vi "(SubVI) Cut Unfold and Fold Startpoint_YCC.vi"(7 "number to cut":i32=15, 8 "Folded-Force in":dbl[](array[numeric]), 9 "Folded-xDNA in":dbl[](array[numeric]), 10 "Unfolded-Force":dbl[](array[numeric]), 11 "Unfolded-xDNA":dbl[](array[numeric])) -> (0 "Folded-Force":dbl[](array[numeric]), 1 "Folded-xDNA":dbl[](array[numeric]), 2 "Unfolded-Force":dbl[](array[numeric]), 3 "Unfolded-xDNA":dbl[](array[numeric]))   [LabVIEW 2014]
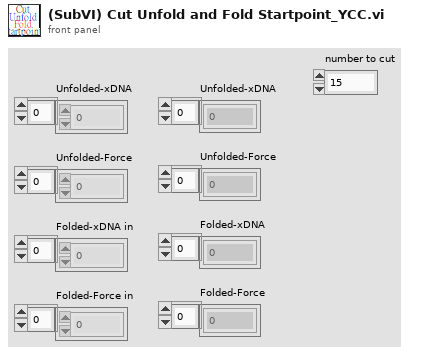
[diagram p1: front panel]
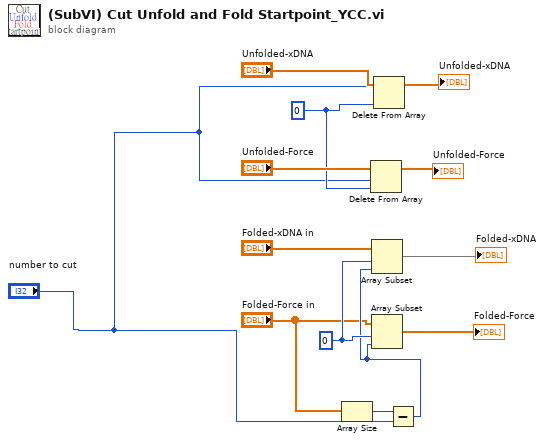
[diagram p0: block diagram]
diagram:
  w11 = 0 ("index")
  w3 = 0 ("index")
  n1 = Array Size(array="Folded-Force in") -> (size(s)=w9:i32)
  n2 = Delete From Array(array="Unfolded-Force", length="number to cut", index=w3) -> (array with subset deleted=→"Unfolded-Force":dbl[])  [unwired: 1 out]
  n3 = Delete From Array(array="Unfolded-xDNA", length="number to cut", index=w3) -> (array with subset deleted=→"Unfolded-xDNA":dbl[])  [unwired: 1 out]
  n4 = Subtract(x=w9, y="number to cut") -> (x-y=w10:i32)
  n5 = Array Subset(array="Folded-xDNA in", index=w11, length=w10) -> (→"Folded-xDNA":dbl[])
  n6 = Array Subset(array="Folded-Force in", index=w11, length=w10) -> (→"Folded-Force":dbl[])
